vi "Try Register API.vi"(8 "error in (no error)":errorcluster, 11 "Task in":refnum<class "Task.lvclass">) -> (0 "error out":errorcluster, 3 "Task out":refnum<class "Task.lvclass">)   [LabVIEW 2020, in "Volatus.lvlib" / "Task.lvclass"]
uses:
  Task.lvclass
  C:/Program Files (x86)/National Instruments/LabVIEW 2020/vi.lib/ActorFramework/Actor/Actor.lvclass
  Task.lvclass/Task.ctl
  <vilib>/ActorFramework/Actor/Actor.lvclass/Actor.ctl
  APIRegistrationHandler Messages/Register API Msg/Register API Msg.lvclass/Register API Msg.ctl
  <vilib>/ActorFramework/Message Enqueuer/Message Enqueuer.lvclass/Message Enqueuer.ctl
  <vilib>/ActorFramework/Message Enqueuer/Enqueue.vi
  APIRegistrationHandler Messages/Register API Msg/Register API Msg.lvclass
  C:/Program Files (x86)/National Instruments/LabVIEW 2020/vi.lib/ActorFramework/Message/Message.lvclass
  <vilib>/ActorFramework/Message Priority Queue/Priority Enqueue.vi
  <vilib>/ActorFramework/Actor/Actor.lvclass
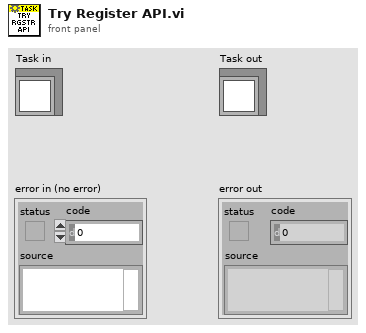
[diagram p1: front panel]
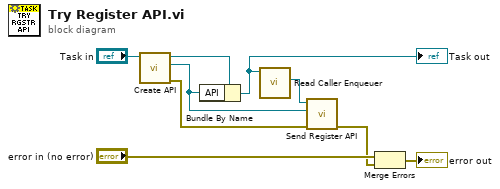
[diagram p0: block diagram]
diagram:
  n1 = call "Create API.vi"("Task in"="Task in") -> ("error out"=w1:errorcluster, "API"=w3:refnum<class "API.lvclass">, "Task out"=w2:refnum<class "Task.lvclass">)  [unwired: 8 in]
  n2 = Bundle By Name(cluster=w2, "API"=w3) -> (w8:refnum<class "Task.lvclass">)
  "Task out" <- w8
  n3 = call <vilib>:"Read Caller Enqueuer.vi"("Actor"=w8) -> ("Caller Enqueuer"=w5:refnum<class "Message Enqueuer.lvclass">)  [unwired: 10 in]
  n4 = call "Send Register API.vi"("error in (no error)"=w1, "API"=w3, "Message Enqueuer"=w5) -> ("error out"=w6:errorcluster)  [unwired: 7 in, 1 out]
  n5 = Merge Errors("error in (no error)", w6) -> (→"error out":errorcluster)
